vi "test3.vi"() -> ()   [LabVIEW 2014]
panel:
  in  "?":bool
  out "L":bool
  in  "A":bool
  in  "B":bool
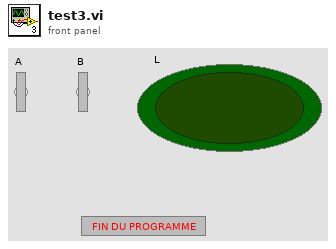
[diagram p1: front panel]
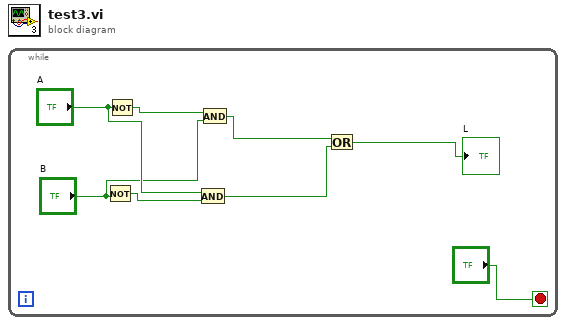
[diagram p0: block diagram]
diagram:
  n1 = while {
    stop <- "?" stop-if-true
    n2 = Not(x="B") -> (.not. x?=w5:bool)
    n3 = Not(x="A") -> (.not. x?=w8:bool)
    n4 = And(x="A", y=w5) -> (x .and. y?=w1:bool)
    n5 = And(x=w8, y="B") -> (x .and. y?=w7:bool)
    n6 = Or(x=w7, y=w1) -> (x .or. y?=→"L":bool)
  }
